vi "Get or Add WorksheetPart.vi"(8 "error in":errorcluster, 10 "Sheet Name":string, 11 "SpreadsheetDoc in":refnum<k24>) -> (0 "error out":errorcluster, 2 "WorksheetPart":refnum<k24>, 3 "SpreadsheetDoc out":refnum<k24>)   [LabVIEW 2019, in "Open Xml.lvlib"]
uses:
  Open Xml.lvlib
  D:/git/Open-Xml-LabVIEW/Source/DocumentFormat.OpenXml.dll
  DocumentFormat.OpenXml.dll
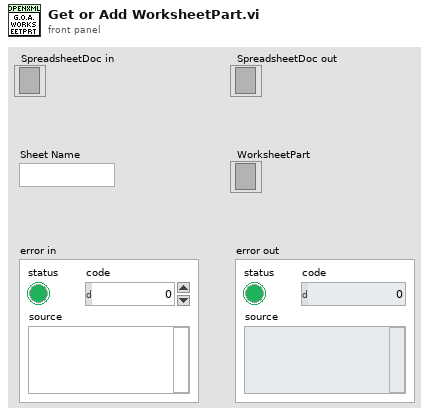
[diagram p1: front panel]
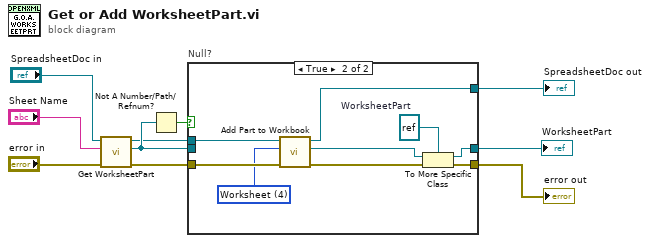
[diagram p0: block diagram]
diagram:
  n1 = call "Get WorksheetPart.vi"("error in"="error in", "Sheet Name"="Sheet Name", "SpreadsheetDoc in"="SpreadsheetDoc in") -> ("error out"=w6:errorcluster, "WorksheetPart"=w5:refnum<k24>, "SpreadsheetDoc out"=w2:refnum<k24>)  [unwired: 5 in, 1 out]
  n2 = Not A Number/Path/Refnum?(number/path/refnum=w5) -> (NaN/Path/Refnum?=w4:bool)
  n3 = case "Null?" shown="True" w4 {
    tunnel: [w12 w20] -> w10
    tunnel: [w13 w18] -> w9
    tunnel: w2 -> [w11 w17]
    tunnel: [w11 w16] -> w8
    tunnel: w6 -> [w13 w15]
    tunnel: w5 -> [w12 _]
    frame False {
    }
    frame True {
      w14 = 4 items=["Connections", "PivotTableCacheDefinition", "PivotTableCacheRecords", "SharedString", "Worksheet", "WorkbookStyles"] ("PartType")
      w21 = refnum<k24> refnum  # WorksheetPart
      n4 = call "Add Part to Workbook.vi"("error in"=w15, "PartType"=w14, "SpreadsheetDoc in"=w17) -> ("error out"=w19:errorcluster, "OpenXmlPart"=w22:refnum<k24>, "SpreadsheetDoc out"=w16:refnum<k24>)  [unwired: 6 in]
      n5 = To More Specific Class(target class=w21, reference=w22, error in=w19) -> (specific class reference=w20:refnum<k24>, error out=w18:errorcluster)
    }
  }
  "WorksheetPart" <- w10
  "error out" <- w9
  "SpreadsheetDoc out" <- w8
